vi "Real Time Doppler Trigger working copy.vi"() -> ()   [LabVIEW 2022 SP3]
doc: "Performs real-time Joint Time Frequency Analysis (JTFA) using Point By Point STFT. The signal is simulated by a sine wave plus Gaussian noise."
uses:
  <vilib>/DAQmx/read.llb/DAQmx Read (Analog 1D DBL 1Chan NSamp).vi
  <vilib>/measure/mamon.llb/Waveform Peak Detection for N Chan.vi
  <vilib>/DAQmx/miscellaneous.llb/DAQmx Fill In Error Info.vi
  ScanningControl/Motion Controllers/-MotionRoutines/MotionGlobals.vi
  <resource>/objmgr/daqmx.rc
  <vilib>/gmath/NI_Gmath.lvlib
  <vilib>/measure/NI_MAPro.lvlib
  <vilib>/ptbypt/NI_PtbyPt.lvlib
panel:
  in  "Doppler Envelope Thresh":dbl=5.0
  in  "STFT Threshold":dbl=0.1
  out "Boolean":bool
  out "Default Num samples 2":dbl=5.0
  out "Doppler envelope":cluster{"Filtered x":dbl, "Filtered x":dbl}[](graph)=[{"Filtered x"=7.088088524907631, "Filtered x"=0.0}, {"Filtered x"=6.960621715402169, "Filtered x"=0.0}, {"Filtered x"=6.831524242593062, "Filtered x"=0.0}, {"Filtered x"=6.701135569871356, "Filtered x"=0.0}, {"Filtered x"=6.569707789620943, "Filtered x"=0.0}]
  in  "Num samples to read":i32=256
  in  "window info":cluster{"type":u32, "window length":u32}={"type"=2, "window length"=128} {"window length" format="%0.0f"; "type" format="%0.0f"}
  in  "time-freq sampling":cluster{"time steps":i32, "freq bins":i32}={"time steps"=64, "freq bins"=128} {"freq bins" format="%0.0f"}
  out "DAQ error":errorcluster
  out "Default Num samples":dbl=1024.0
  in  "DAQmx Task Name":refnum<k21>="DopplerI"
  out "fs":dbl=48076.92307692308
  out "Moving STFT":dbl[][](graph)=[[0.7758616192820993, 0.7552502788970572, 0.9463820257089955, 0.8858805585579104, 0.41291286730537874, 0.0846200183961221, 0.0033730286577622923, 0.006612139288461409, 0.0061476574094778535, 0.008190982767285285, 0.0038637013677402425, 0.009323332825878416, 0.002152466015687241, 0.0030963054709158165, 0.0024672832898785095, 0.0023731613687951545, 0.0007461028969798001, 0.0027241172448886275, 0.0007889732229935198, 0.0014710127321130935, 0.0007747511525448659, 0.00134333967607672, 0.00046264618181361965, 0.0012934901813567972, 0.0006135588728345639, 0.0011098716208680023, 0.0003597614336957922, 0.0011513092030117193, 0.00044026525711584973, 0.0005482299938310904, 0.00019922747092289048, 0.00042516256759290186, 0.00014348822765209636, 0.0006384106412564417, 0.00018839635343866456, 0.0005009048377563736, 0.00015351963163361918, 0.00022647630580307384, 5.171516780249453e-05, 0.0007125501620546158, 0.0010338594575594702, 0.0012678148508367616, 0.00039349041938880827, 0.0005571563247911949, 0.00031747899936686574, 0.0005303977649655228, 0.00021873342131623847, 0.0006238507049128933, 0.00028354306307848946, 0.0004731963960631171, 0.00021273063424381405, 0.0004403060870093573, 0.00018001474357166595, 0.0004164047287170246, 0.00020510794078082529, 0.00040077012927002524, 0.00015897204111342412, 0.0004242637173948257, 0.00018146168543039127, 0.0003626254353805943, 0.00018164060279937853, 0.0003952581390912309, 0.00015661445419220554, 0.00038510049394619453], [29.560874980134702, 12.18944245551451, 1.2702570450477528, 1.4771907539601914, 1.6461188266827844, 0.07922282968681443, 0.002304235497911286, 0.008710788654921421, 0.0034500170920290876, 0.0013577134464296035, 0.002169552551914873, 0.0015369828554716645, 0.0016039201288484191, 0.0012541183475775627, 0.0007945229380734591, 0.0007738223548531382, 0.0003536728258870138, 0.00021325330609596696, 0.00014973728687125623, 5.771218605987644e-05, 3.295961720587466e-07, 7.483357088769246e-05, 0.00012073410578964026, 3.222898285151718e-05, 4.983543838019289e-05, 6.780148751328928e-05, 2.5500533015200685e-05, 5.509256362921087e-05, 8.48013806028995e-05, 5.300957388692363e-05, 5.165949648381474e-05, 0.0001394088599623887, 5.955145554143955e-05, 2.8220475848135158e-05, 3.22925416959254e-05, 1.701716950248667e-05, 1.0656449357450934e-05, 2.1237038358715188e-05, 2.8788747221685852e-05, 0.0008702529564265575, 0.0003466019239319481, 6.00171103144457e-07, 1.7281861701107075e-05, 2.223194685879342e-05, 7.593195298081867e-06, 1.787570593955667e-05, 2.7819768250520294e-05, 9.697921955951008e-06, 1.2588085820729335e-05, 2.2328394614186396e-06, 2.6560582812100254e-07, 2.3785114095582027e-06, 9.938485148411413e-07, 3.6511784998285074e-06, 9.599875461116721e-09, 1.7940878542962293e-06, 9.302418380320412e-06, 1.3120157688988683e-06, 2.514421991124468e-06, 6.856223762437897e-06, 1.1663112864680908e-06, 2.7797805170534537e-06, 1.9410318728121137e-06, 1.1765892998719591e-06], [0.8907972537074527, 14.395958262914487, 8.344629906073713, 2.324608357696733, 0.05990374480942586, 0.007010604410482472, 0.00896410347457491, 0.006344467456556225, 0.0015167238212347382, 0.0021250768658790903, 0.0030740168853338554, 0.0002597908607051017, 0.00042673199464226863, 0.0011389050118589125, 0.0003396791565894723, 0.00026250001892634604, 0.00044049309552212875, 5.728629709288822e-05, 0.0003183398216338738, 0.0003694956690842214, 8.072837749468497e-05, 0.0001188253859321057, 0.00011933854763046513, 0.00028834208288004107, 2.2376525754276138e-05, 0.0002916713518796591, 0.00012116373545037137, 0.00013538554085812355, 3.5821973357350756e-05, 0.00012644128672824556, 2.567652426219146e-05, 0.00018465176862160783, 0.00017915744810452708, 1.6401842552410684e-05, 0.0001512638695533414, 4.6277362072054356e-05, 0.00010377999388927325, 3.457375040657594e-05, 3.3667648028858494e-05, 0.0003729637921222282, 0.0001039219261276297, 7.788872725515117e-05, 3.9716846702827544e-05, 4.1813867493274705e-05, 0.00013089161522761652, 1.8691225422850323e-05, 6.164953510599312e-05, 5.2586854878574615e-05, 2.9531036951931138e-05, 4.303920614436281e-05, 5.240690334776885e-05, 4.945673045165185e-05, 3.176960191142804e-05, 4.1122207310636374e-05, 4.956471000985458e-05, 2.8250397522344502e-05, 6.065625984487329e-05, 4.892507374970653e-05, 2.3065891257059715e-05, 5.438330580107524e-05, 4.312554559465404e-05, 2.8808860138020307e-05, 5.1399461989838496e-05, 4.001582906382082e-05], [18.619912856089975, 16.285121927301727, 0.12297710167253291, 0.9733273111461695, 0.25207442674357544, 0.02980835614037296, 0.008245639335136253, 0.002272752687083841, 0.00353924461111596, 0.0019756116209230326, 0.0005849348384708688, 0.0005348707374887256, 7.549389703453243e-06, 1.8071596509075945e-06, 0.0002445278630391338, 0.00013784625036582975, 5.5800687600630684e-05, 4.8134435761781704e-05, 5.666300033262535e-05, 5.621012952332507e-05, 0.00013050451444471633, 3.010112773133447e-05, 3.2929750937589884e-05, 9.621714041733908e-05, 8.496311684338847e-06, 2.2714394314291495e-05, 3.883995929167459e-05, 1.52156213713623e-05, 1.506419669304899e-05, 4.05263293526373e-05, 4.772462329427735e-05, 6.648368142491165e-05, 0.00014492999601032543, 3.6376410898278603e-06, 4.2939861293991806e-05, 1.0248456683649135e-05, 1.0308248425589834e-05, 6.347915783178811e-06, 7.727144505219963e-05, 8.449122643539573e-05, 5.3127034417916814e-05, 2.1974586066762178e-05, 1.5324398317234736e-05, 3.800784118114265e-05, 2.330269728763723e-05, 1.581936244093772e-05, 6.017857493659411e-06, 1.9227458844400613e-05, 1.0161521646161964e-06, 1.0976820450191384e-05, 9.46560340598065e-06, 9.682420055204577e-06, 5.68422777553608e-06, 3.803645858962153e-05, 1.9161296945624465e-06, 1.0190189817520987e-05, 1.1347894301271295e-05, 8.179139327171507e-06, 2.4662381674841076e-06, 5.899508556158426e-06, 8.09874137397642e-06, 1.114689070570955e-05, 2.998363877900547e-06, 1.4350886132871018e-05], [4.713118012021028, 5.37355591395059, 4.756257717590666, 2.2480994231454443, 0.5978598426056971, 0.08609708043660719, 0.015133394090150992, 0.015701354897715788, 0.009025475048759082, 0.007330186665068654, 0.0007556998508641515, 0.0013046867685186942, 0.0004112759998421367, 0.0012584368181379772, 0.0004863486299785702, 0.001020729251770022, 7.695160425614709e-05, 0.00025578475209463326, 5.544114806583293e-05, 0.00044315463221741456, 0.00014603179093490503, 0.0004680064209717532, 0.0001066368732709842, 0.00037256482312870634, 4.407138296193238e-05, 5.618852009103928e-05, 4.609635627187632e-06, 9.156383144275654e-05, 5.148393446283566e-06, 0.00010648221576575437, 1.9888416953841376e-06, 4.038429126314003e-05, 3.560986568978737e-05, 0.00018676288955373169, 3.368000292904106e-05, 0.00013968496806861054, 1.2549508921088358e-05, 8.482179755181282e-05, 4.189095873464004e-05, 7.795734329354568e-05, 9.129026611250584e-05, 1.606307730287014e-05, 9.630794415080201e-06, 1.2506824880394625e-05, 2.8672471397917286e-05, 6.154959791409237e-05, 1.0094563109750752e-05, 6.065507883368708e-05, 6.401331216869644e-07, 3.888178507065707e-05, 2.0845065258836607e-06, 4.471759426194118e-05, 2.7976039396303857e-06, 5.037421863665822e-05, 6.477484514509946e-07, 2.939282364528865e-05, 2.024036841939181e-06, 3.870964831451266e-05, 2.3370882295555736e-06, 4.5468907681824e-05, 3.504320007570383e-06, 5.129593416742216e-05, 4.489280335832992e-06, 7.811527132994124e-05]]
  in  "stop":bool
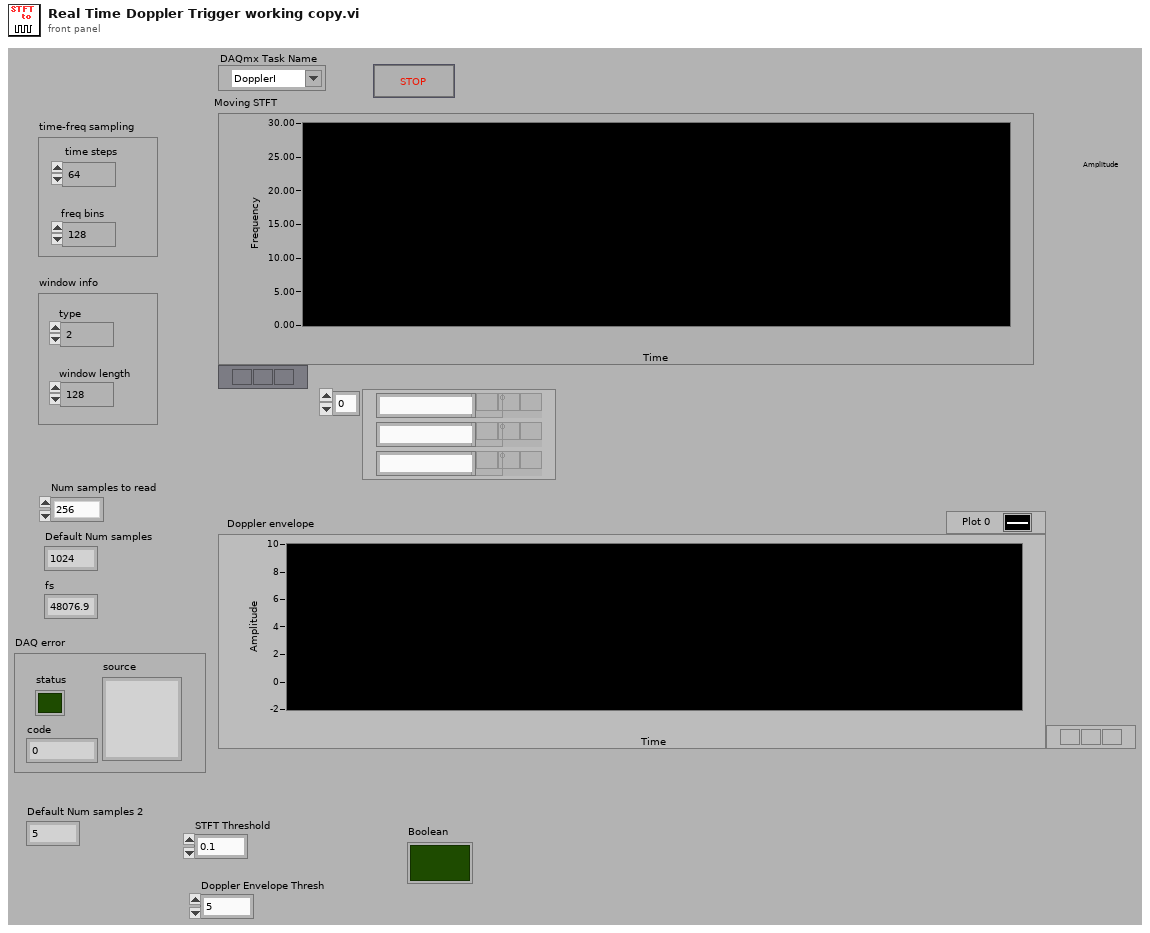
[diagram p1: front panel]
types:
  T1 = enum16{"Lowpass", "Highpass", "Bandpass", "Bandstop"}
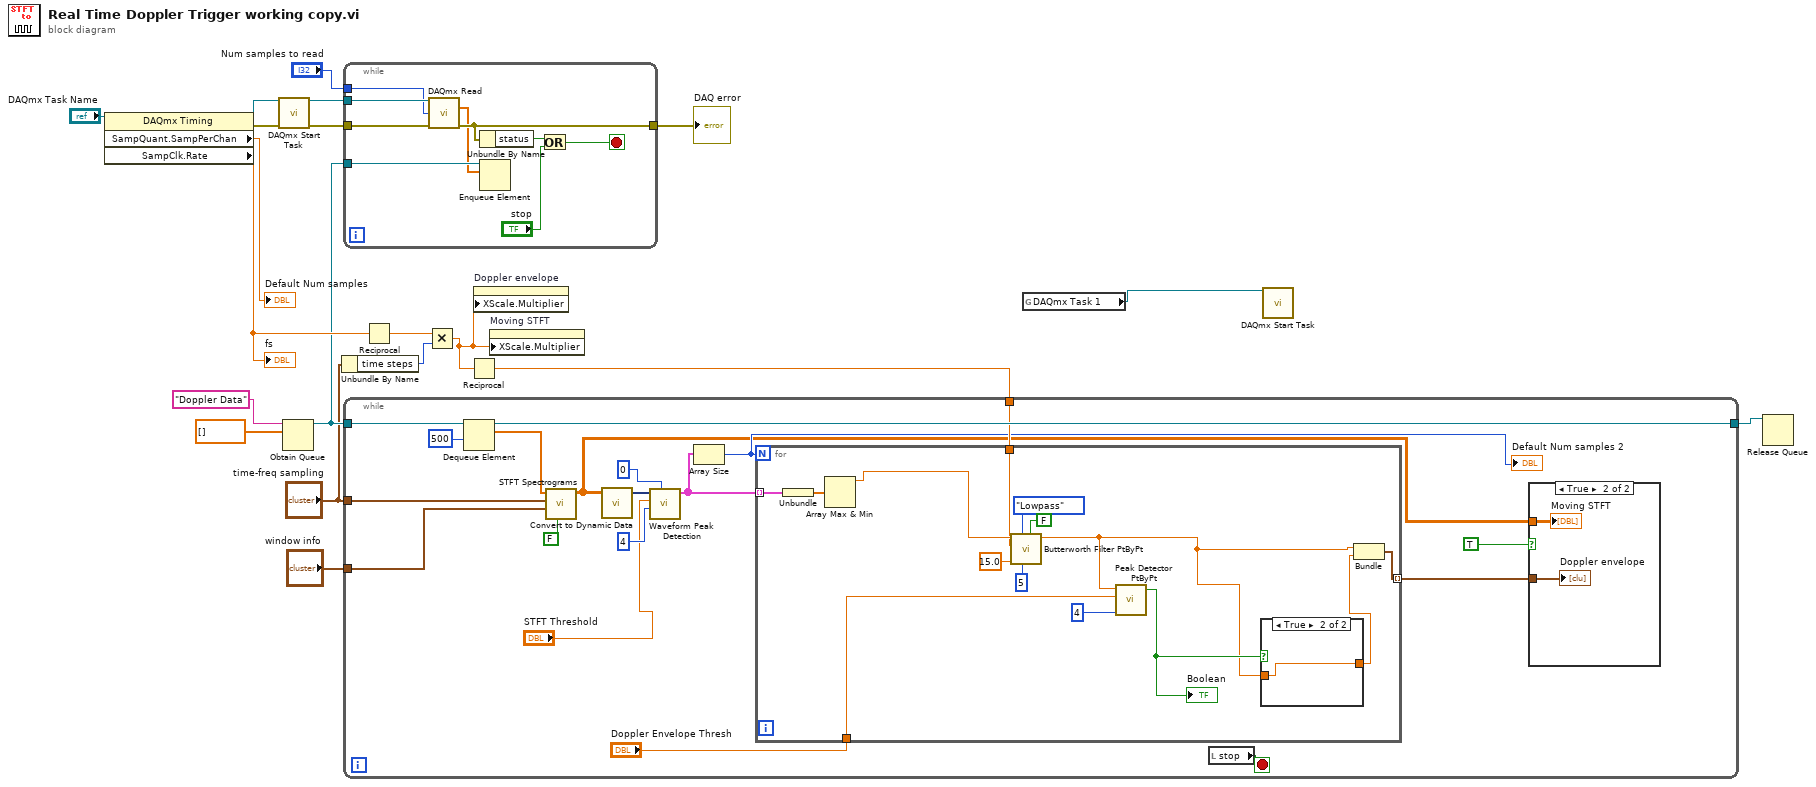
[diagram p0: block diagram]
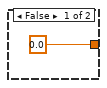
[diagram p3: hidden frame]
diagram:
  n1 = property class="DAQmx Timing"(reference="DAQmx Task Name") -> (reference out=w19:refnum<k21>, error out=w18:errorcluster, "SampQuant.SampPerChan"=→"Default Num samples":dbl, "SampClk.Rate"=w14:dbl)  [unwired: 1 in]
  "fs" <- w14
  n2 = call <vilib>:"DAQmx Start Task.vi"("task/channels in"=w19, "error in"=w18) -> ("task out"=w17:refnum<k21>, "error out"=w16:errorcluster)  [unwired: 12 out]
  n3 = Obtain Queue(name (unnamed)="Doppler Data", element data type=dbl[] [] ("Y")) -> (queue out=w12:refnum<queue>)  [unwired: 3 in, 2 out]
  n4 = Unbundle By Name("time-freq sampling") -> ("time steps"=w4:i32)
  n5 = while {
    tunnel: w17 -> [w29]
    tunnel: [w23] -> w20
    tunnel: w16 -> [w28]
    tunnel: w12 -> [w27]
    tunnel: "Num samples to read" -> [w26]
    stop <- w24 stop-if-true
    n6 = call-poly <vilib>:"DAQmx Read.vi"("task/channels in"=w29, "number of samples per channel"=w26, "error in"=w28) -> ("data"=w21:dbl[], "error out"=w23:errorcluster)  [unwired: 11 out]
    n7 = Unbundle By Name(w23) -> ("status"=w22:bool)
    n8 = Enqueue Element(queue=w27, element=w21) -> ()  [unwired: 1 in, 4 out]
    n9 = Or(x=w22, y="stop") -> (x .or. y?=w24:bool)
  }
  "DAQ error" <- w20
  n10 = Reciprocal(x=w14) -> (1/x=w5:dbl)
  n11 = Multiply(x=w5, y=w4) -> (x*y=w2:dbl)
  n12 = Reciprocal(x=w2) -> (1/x=w3:dbl)
  n13 = while {
    tunnel: w12 -> [w43]
    tunnel: "time-freq sampling" -> [w48]
    tunnel: "window info" -> [w47]
    tunnel: [w42] -> w9
    tunnel: w3 -> [w36]
    stop <- w37 stop-if-true
    n14 = Dequeue Element(queue=w43, timeout in ms (-1)=500) -> (queue out=w42:refnum<queue>, element=w45:dbl[])  [unwired: 1 in, 2 out]
    n15 = call <vilib>:"STFT Spectrograms.vi"("energy conservation?"=FALSE, "window info"=w47, "time-freq sampling info"=w48, "X"=w45) -> ("STFT Spectrogram {X}"=w32:dbl[][])  [unwired: 2 in, 5 out]
    n16 = call "Convert to Dynamic Data"("2D Array"=w32) -> ("Dynamic Data Type"=w38:dynamicdata)  [unwired: 3 out]
    n17 = call-poly <vilib>:"Waveform Peak Detection.vi"("peaks/valleys"=u32 0 ("milliseconds to wait"), "width"=u32 4 ("milliseconds to wait"), "threshold"="STFT Threshold", "Signals In"=w38) -> ("Locations"=w41:cluster{"Locations":dbl[]}[])  [unwired: 3 in, 4 out]
    n18 = Array Size(array=w41) -> (size(s)=w33:i32)
    "Default Num samples 2" <- w33
    n19 = for {
      N: w33 -> [_]
      tunnel: w41 -> [w55] mode=indexing
      tunnel: w36 -> [w59]
      tunnel: "Doppler Envelope Thresh" -> [w56]
      tunnel: [w51] -> w30 mode=indexing
      n20 = Unbundle(w55) -> ("Locations"=w64:dbl[])
      n21 = Array Max & Min(array=w64) -> (max value=w62:dbl)  [unwired: 3 out]
      n22 = call <vilib>:"Butterworth Filter PtByPt.vi"("initialize"=FALSE, "order"=5, "filter type"=T1."Lowpass", "low cutoff freq: fl"=15.0, "sampling freq: fs"=w59, "x"=w62) -> ("Filtered x"=w53:dbl)  [unwired: 1 in, 3 out]
      n23 = call <vilib>:"Peak Detector PtByPt.vi"("x"=w53, "threshold peak"=w56, "width"=u32 4 ("milliseconds to wait")) -> ("peak"=w54:bool)  [unwired: 2 in, 2 out]
      "Boolean" <- w54
      n24 = case shown="True" w54 {
        tunnel: [0.0 ("milliseconds to wait") w66] -> w52
        tunnel: w53 -> [_ w66]
        frame False {
        }
        frame True {
        }
      }
      n25 = Bundle("Filtered x"=w53, "Filtered x"=w52) -> (w51:cluster{"Filtered x":dbl, "Filtered x":dbl})  [unwired: 1 out]
    }
    n26 = local read "stop"() -> (w37:bool)
    n27 = case shown="True" TRUE {
      tunnel: w32 -> [_ w50]
      tunnel: w30 -> [_ w49]
      frame False {
      }
      frame True {
        "Moving STFT" <- w50
        "Doppler envelope" <- w49
      }
    }
  }
  n28 = property on="Doppler envelope" class="WFChart (strict)"("XScale.Multiplier"=w2) -> ()  [unwired: 2 in, 2 out]
  n29 = property on="Moving STFT" class="IntChart (strict)"("XScale.Multiplier"=w2) -> ()  [unwired: 2 in, 2 out]
  n30 = global read "MotionGlobals.vi" "DAQmx Task 1"() -> (w1:refnum<k21>)
  n31 = call <vilib>:"DAQmx Start Task.vi"("task/channels in"=w1) -> ()  [unwired: 1 in, 14 out]
  n32 = Release Queue(queue=w9) -> ()  [unwired: 1 in, 4 out]
